vi "Connection Manager.vi"(11 "Custom Outputs":string[](array[string])) -> ()   [LabVIEW 2020]
uses:
  Type Defs/PXISlot XControl/PXISlot.xctl
  Type Defs/PXISlot XControl/Connector Type.ctl
  <vilib>/Utility/config.llb/Read Key (Boolean).vi
  <vilib>/Utility/config.llb/Write Key (Boolean).vi
  <vilib>/Utility/config.llb/NI_LVConfig.lvlib
panel:
  in  "Breakout box type":enum32{"BNC-2090", "BNC-2110"}(radio)
  in  "Hide unused":bool
  in  "Exit":bool
  in  "Save":bool
  in  "Slot3":T3(xcontrol) caption="Slot 3"
  in  "Slot2":T3(xcontrol) caption="Slot 2"
  in  "Slot9":T3(xcontrol) caption="Slot 3"
  in  "Slot8":T3(xcontrol) caption="Slot 3"
  in  "Slot7":T3(xcontrol) caption="Slot 3"
  in  "Slot6":T3(xcontrol) caption="Slot 3"
  in  "Slot5":T3(xcontrol) caption="Slot 5"
  in  "Slot4":T3(xcontrol) caption="Slot 3"
  # "Inputs"
  # "Outputs"
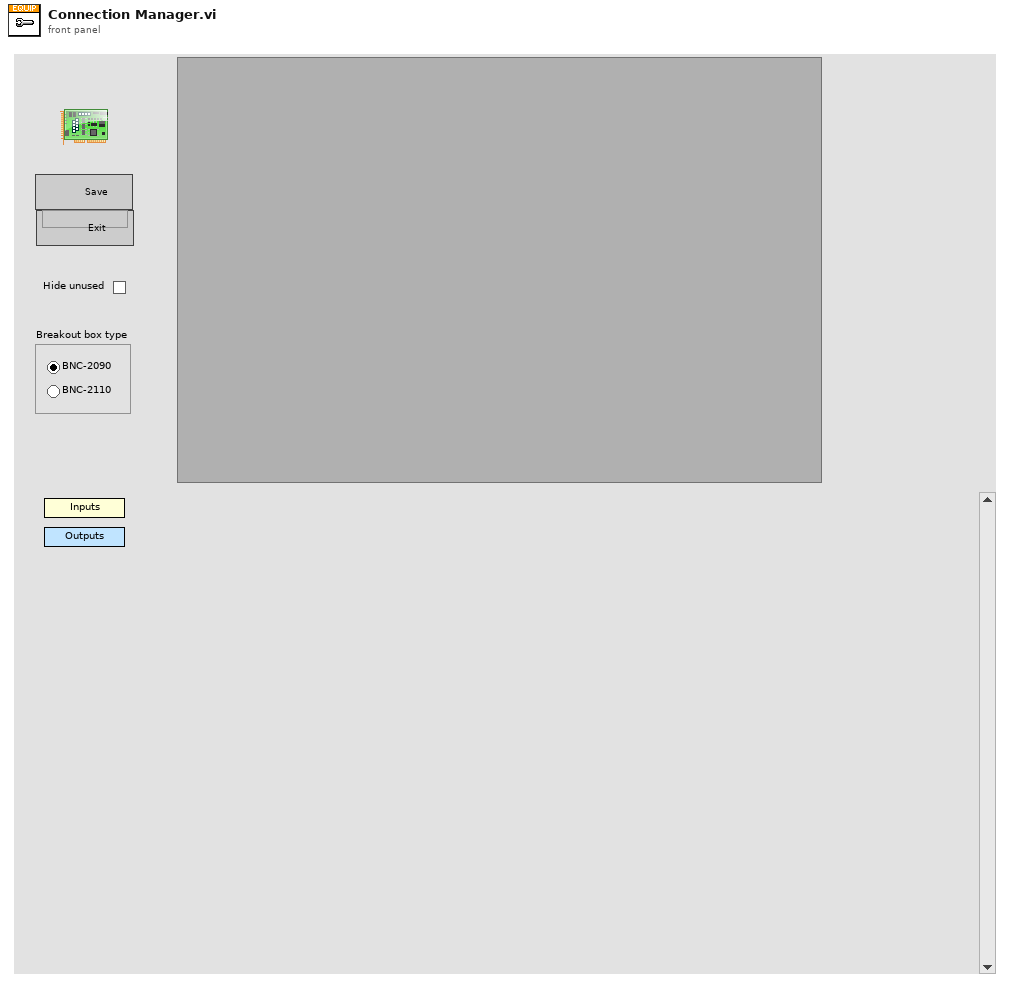
[diagram p1: front panel]
types:
  T1 = typedef "Output sources.ctl" = u16
  T2 = typedef "Input sources.ctl" = u16
  T3 = cluster{"Output sources":T1[], "Input sources":T2[]}
  T4 = typedef "Connector Type.ctl" = enum16{"None", "PXI-4461", "BNC-2110", "BNC-2090", "PXIe-4463", "PXIe-4464"}
  T5 = typedef "NI_LVConfig.lvlib/Config Data RefNum.ctl" = refnum<k1>
  T6 = cluster{"DAQChan to PhysDev":i32[][], "PhysDev to DAQChan":i32[][]}
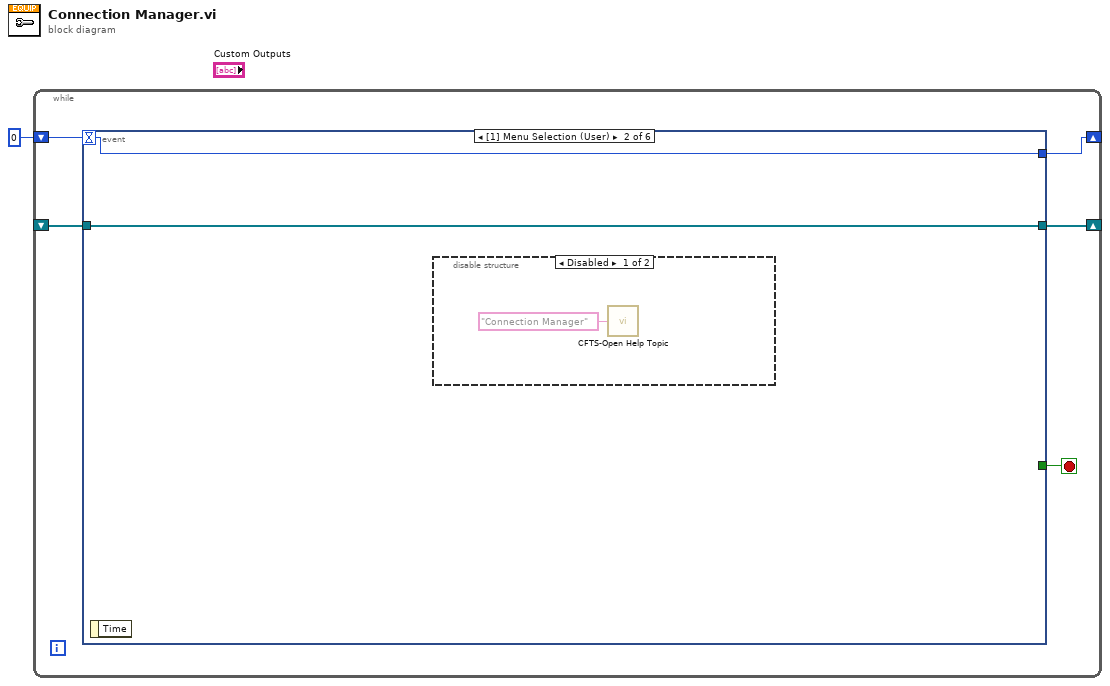
[diagram p0: block diagram]
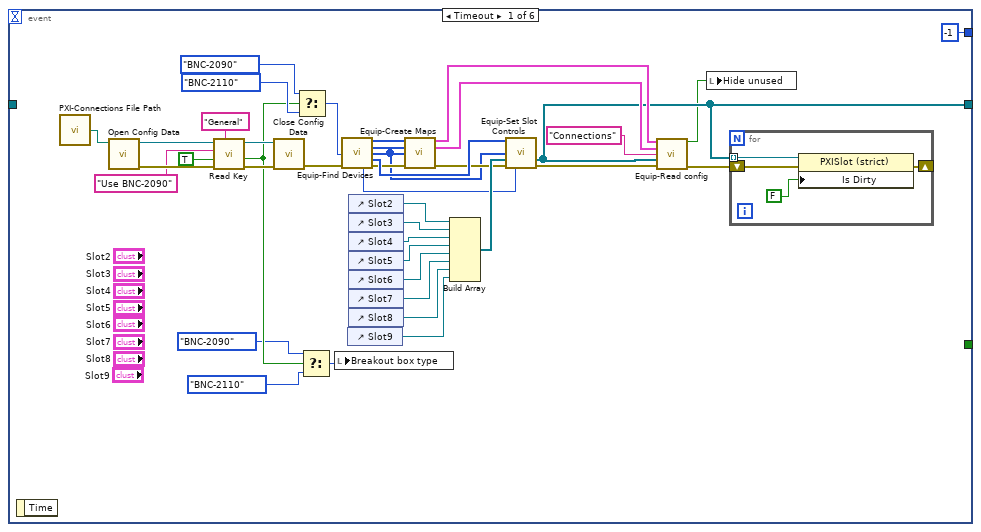
[diagram p2: hidden frame]
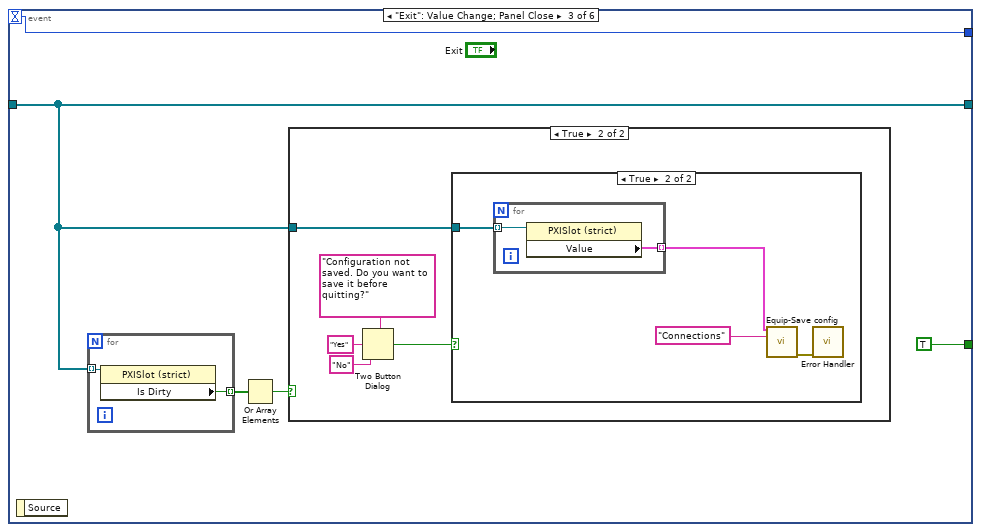
[diagram p4: hidden frame]
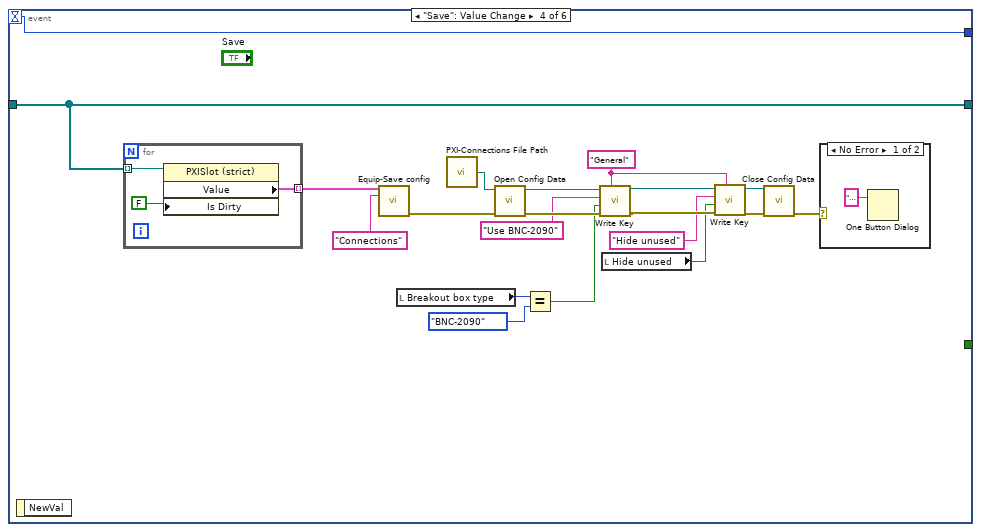
[diagram p7: hidden frame]
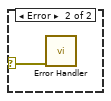
[diagram p8: hidden frame]
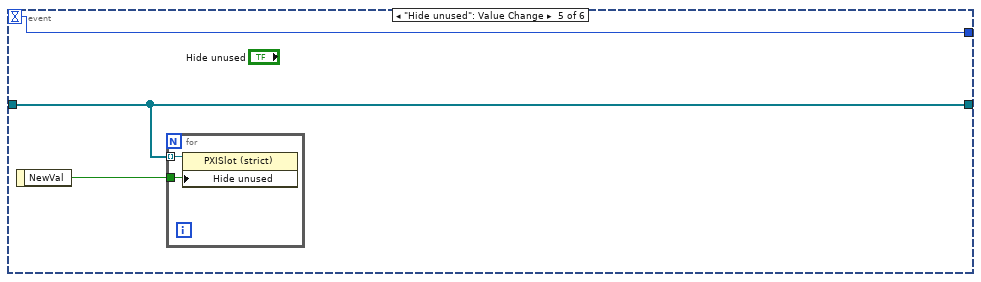
[diagram p9: hidden frame]
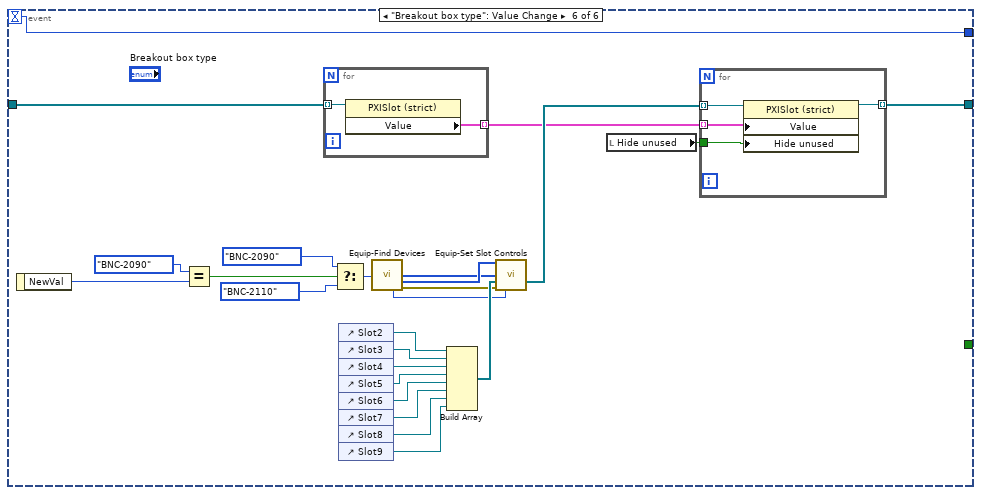
[diagram p10: hidden frame]
diagram:
  n1 = while {
    shift-right: [w4] -> _
    shift-left: 0 -> [w5]
    shift-right: [w3] -> _
    shift-left: _ -> [w2]
    stop <- w6 stop-if-true
    n2 = event shown="[1] Menu Selection (User)" {
      selector: _ -> [_ _ _ _ _ _]
      dyn-events: _ -> [_ _ _ _ _ _]
      timeout: w5 -> [_ w52 w55 w90 w98 w126]
      tunnel: [_ _ TRUE _ _ _] -> w6
      tunnel: [-1 w52 w55 w90 w98 w126] -> w4
      tunnel: [w30 w51 w54 w88 w97 w108] -> w3
      tunnel: w2 -> [_ w51 w54 w88 w97 w111]
      event Timeout {
        n3 = event-data() -> ()  [unwired: 1 in, 1 out]
        n4 = call "PXI-Connections File Path.vi"() -> ("Path"=w7:path)  [unwired: 1 in]
        n5 = call <vilib>:"Open Config Data.vi"("configuration file path"=w7) -> ("error out"=w27:errorcluster, "refnum"=w28:T5)  [unwired: 8 in, 1 out]
        n6 = call-poly <vilib>:"Read Key.vi"("section"="General", "error in (no error)"=w27, "default value"=TRUE, "key"="Use BNC-2090", "refnum"=w28) -> ("error out"=w23:errorcluster, "value"=w17:bool, "refnum out"=w22:T5)  [unwired: 3 in, 1 out]
        n7 = call <vilib>:"Close Config Data.vi"("error in (no error)"=w23, "refnum"=w22) -> ("error out"=w19:errorcluster)  [unwired: 8 in, 1 out]
        n8 = Select(t=Connector_Type."BNC-2090" ("16-bit breakout"), s=w17, f=Connector_Type."BNC-2110" ("16-bit breakout")) -> (s? t:f=w20:T4)
        n9 = Select(t=enum32{"BNC-2090", "BNC-2110"}."BNC-2090", s=w17, f=enum32{"BNC-2090", "BNC-2110"}."BNC-2110" ("Breakout box type")) -> (s? t:f=w14:enum32{"BNC-2090", "BNC-2110"})
        n10 = local write "Breakout box type"(w14) -> ()
        n11 = call "Equip-Find Devices.vi"("16-bit breakout"=w20, "error in (no error)"=w19) -> ("Num AO"=w35:i32[], "Num AI"=w36:i32[], "Slot Num"=w11:u32[], "connector types"=w41:T4[], "Trigger Slot"=w13:i32, "error out"=w37:errorcluster)  [unwired: 8 in]
        n12 = control-ref of="Slot9"() -> (w8:refnum<vi>)
        n13 = control-ref of="Slot2"() -> (w33:refnum<vi>)
        n14 = control-ref of="Slot3"() -> (w34:refnum<vi>)
        n15 = control-ref of="Slot4"() -> (w44:refnum<vi>)
        n16 = control-ref of="Slot5"() -> (w45:refnum<vi>)
        n17 = control-ref of="Slot6"() -> (w29:refnum<vi>)
        n18 = control-ref of="Slot7"() -> (w10:refnum<vi>)
        n19 = control-ref of="Slot8"() -> (w9:refnum<vi>)
        n20 = call "Equip-Create Maps.vi"("Num AO"=w35, "Num AI"=w36, "Slot Num"=w11, "error in (no error)"=w37) -> ("AO Map"=w32:T6, "AI Map"=w31:T6, "error out"=w38:errorcluster)  [unwired: 9 in]
        n21 = Build Array(w33, w34, w44, w45, w29, w10, w9, w8) -> (w40:refnum<vi>[])
        n22 = call "Equip-Set Slot Controls.vi"("connector types"=w41, "Slot Num"=w11, "slot ctl refs"=w40, "error in (no error)"=w38, "Trigger Slot"=w13) -> ("slot ctl refs out"=w30:refnum<vi>[], "error out"=w42:errorcluster)  [unwired: 9 in]
        n23 = call "Equip-Read config.vi"("AO Map"=w32, "AI Map"=w31, "config name"="Connections", "slot ctl refs"=w30, "error in (no error)"=w42) -> ("Hide unused?"=w12:bool, "error out"=w39:errorcluster)  [unwired: 9 in]
        n24 = local write "Hide unused"(w12) -> ()
        n25 = for {
          tunnel: w30 -> [w50] mode=indexing
          shift-right: [w48] -> _
          shift-left: w39 -> [w49]
          n26 = property class="PXISlot (strict)"(reference=w50, error in=w49, "Is Dirty"=FALSE) -> (error out=w48:errorcluster)  [unwired: 1 out]
        }
      }
      event Menu Selection (User) {
        n27 = event-data() -> ()  [unwired: 1 in, 1 out]
        n28 = disable-structure shown="Disabled" {
          frame Disabled {
            n29 = call "CFTS-Open Help Topic.vi"("Topic Keyword"="Connection Manager") -> ()  [unwired: 14 in, 1 out]
          }
          frame Enabled {
          }
        }
      }
      event "Exit": Value Change; Panel Close {
        n30 = event-data() -> ()  [unwired: 1 in, 1 out]
        n31 = for {
          tunnel: w54 -> [w60] mode=indexing
          tunnel: [w59] -> w57 mode=indexing
          n32 = property class="PXISlot (strict)"(reference=w60) -> ("Is Dirty"=w59:bool)  [unwired: 1 in, 2 out]
        }
        n33 = Or Array Elements(Boolean array=w57) -> (logical OR=w56:bool)
        n34 = case shown="True" w56 {
          tunnel: w54 -> [_ w61]
          frame False {
          }
          frame True {
            n35 = Two Button Dialog(message="Configuration not saved. Do you want to save it before quitting?", 1:"No" ("F button name (\"Cancel\")"), 2:"Yes" ("T button name (\"OK\")")) -> (T button?=w62:bool)
            n36 = case shown="True" w62 {
              tunnel: w61 -> [_ w67]
              frame False {
              }
              frame True {
                n37 = for {
                  tunnel: w67 -> [w71] mode=indexing
                  tunnel: [w70] -> w66 mode=indexing
                  n38 = property class="PXISlot (strict)"(reference=w71) -> ("Value"=w70:T3)  [unwired: 1 in, 2 out]
                }
                n39 = call "Equip-Save config.vi"("Slots"=w66, "config name"="Connections") -> ("error out"=w69:errorcluster)  [unwired: 13 in]
                n40 = call "Error Handler.vi"("error in (no error)"=w69) -> ()  [unwired: 13 in, 2 out]
              }
            }
          }
        }
      }
      event "Save": Value Change {
        w80 = "General" ("section")
        n41 = event-data() -> ()  [unwired: 1 in, 1 out]
        n42 = for {
          tunnel: w88 -> [w96] mode=indexing
          tunnel: [w94] -> w89 mode=indexing
          n43 = property class="PXISlot (strict)"(reference=w96, "Is Dirty"=FALSE) -> ("Value"=w94:T3)  [unwired: 1 in, 2 out]
        }
        n44 = call "Equip-Save config.vi"("Slots"=w89, "config name"="Connections") -> ("error out"=w84:errorcluster)  [unwired: 13 in]
        n45 = local read "Breakout box type"() -> (w83:enum32{"BNC-2090", "BNC-2110"})
        n46 = call "PXI-Connections File Path.vi"() -> ("Path"=w73:path)  [unwired: 1 in]
        n47 = call <vilib>:"Open Config Data.vi"("error in (no error)"=w84, "configuration file path"=w73) -> ("error out"=w86:errorcluster, "refnum"=w87:T5)  [unwired: 7 in, 1 out]
        n48 = Equal?(x=w83, y=enum32{"BNC-2090", "BNC-2110"}."BNC-2090") -> (x = y?=w81:bool)
        n49 = call-poly <vilib>:"Write Key.vi"("section"=w80, "error in (no error)"=w86, "value"=w81, "key"="Use BNC-2090", "refnum"=w87) -> ("error out"=w77:errorcluster, "refnum out"=w76:T5)  [unwired: 4 in, 1 out]
        n50 = local read "Hide unused"() -> (w74:bool)
        n51 = call-poly <vilib>:"Write Key.vi"("section"=w80, "error in (no error)"=w77, "value"=w74, "key"="Hide unused", "refnum"=w76) -> ("error out"=w78:errorcluster, "refnum out"=w79:T5)  [unwired: 4 in, 1 out]
        n52 = call <vilib>:"Close Config Data.vi"("error in (no error)"=w78, "refnum"=w79) -> ("error out"=w72:errorcluster)  [unwired: 8 in, 1 out]
        n53 = case shown="No Error" w72 {
          selector: w72 -> [_ w93]
          frame No Error {
            n54 = One Button Dialog(message="Hardware configuration saved.") -> ()  [unwired: 1 in, 1 out]
          }
          frame Error {
            n55 = call "Error Handler.vi"("error in (no error)"=w93) -> ()  [unwired: 13 in, 2 out]
          }
        }
      }
      event "Hide unused": Value Change {
        n56 = event-data() -> ("NewVal"=w99:bool)  [unwired: 1 in]
        n57 = for {
          tunnel: w97 -> [w101] mode=indexing
          tunnel: w99 -> [w100]
          n58 = property class="PXISlot (strict)"(reference=w101, "Hide unused"=w100) -> ()  [unwired: 1 in, 2 out]
        }
      }
      event "Breakout box type": Value Change {
        n59 = event-data() -> ("NewVal"=w114:enum32{"BNC-2090", "BNC-2110"})  [unwired: 1 in]
        n60 = Equal?(x=enum32{"BNC-2090", "BNC-2110"}."BNC-2090", y=w114) -> (x = y?=w112:bool)
        n61 = for {
          tunnel: w111 -> [w132] mode=indexing
          tunnel: [w131] -> w109 mode=indexing
          n62 = property class="PXISlot (strict)"(reference=w132) -> ("Value"=w131:T3)  [unwired: 1 in, 2 out]
        }
        n63 = Select(t=Connector_Type."BNC-2090" ("16-bit breakout"), s=w112, f=Connector_Type."BNC-2110" ("16-bit breakout")) -> (s? t:f=w117:T4)
        n64 = control-ref of="Slot2"() -> (w120:refnum<vi>)
        n65 = control-ref of="Slot3"() -> (w121:refnum<vi>)
        n66 = control-ref of="Slot4"() -> (w124:refnum<vi>)
        n67 = control-ref of="Slot5"() -> (w125:refnum<vi>)
        n68 = control-ref of="Slot6"() -> (w119:refnum<vi>)
        n69 = control-ref of="Slot7"() -> (w105:refnum<vi>)
        n70 = control-ref of="Slot8"() -> (w104:refnum<vi>)
        n71 = control-ref of="Slot9"() -> (w103:refnum<vi>)
        n72 = call "Equip-Find Devices.vi"("16-bit breakout"=w117) -> ("Slot Num"=w102:u32[], "connector types"=w123:T4[], "Trigger Slot"=w106:i32, "error out"=w115:errorcluster)  [unwired: 9 in, 2 out]
        n73 = Build Array(w120, w121, w124, w125, w119, w105, w104, w103) -> (w122:refnum<vi>[])
        n74 = call "Equip-Set Slot Controls.vi"("connector types"=w123, "Slot Num"=w102, "slot ctl refs"=w122, "error in (no error)"=w115, "Trigger Slot"=w106) -> ("slot ctl refs out"=w110:refnum<vi>[])  [unwired: 9 in, 1 out]
        n75 = local read "Hide unused"() -> (w107:bool)
        n76 = for {
          tunnel: w110 -> [w130] mode=indexing
          tunnel: w109 -> [w129] mode=indexing
          tunnel: [w128] -> w108 mode=indexing
          tunnel: w107 -> [w127]
          n77 = property class="PXISlot (strict)"(reference=w130, "Value"=w129, "Hide unused"=w127) -> (reference out=w128:refnum<vi>)  [unwired: 1 in, 1 out]
        }
      }
    }
  }
